vi "diagnostic.vi"(10 "Inp":u64) -> (0 "diagnostic3":i32, 1 "diagnostic2":i32, 2 "diagnostic1":i32)   [LabVIEW 2013]
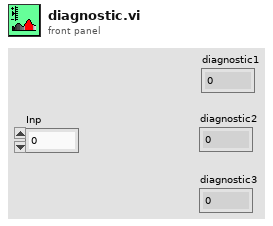
[diagram p1: front panel]
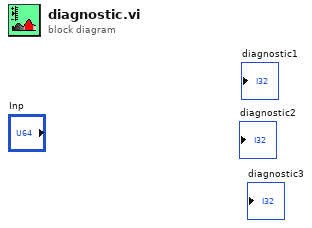
[diagram p0: block diagram]
diagram:
